vi "Update Table with Sensor Data.vi"(0 "Test Table In":string[][](table)=[["", "20"]] caption="Table", 5 "Test Data":dbl[](array[numeric]), 7 "Number of Sensors":i32=7) -> (1 "Current Elapsed":dbl format="%.2g", 2 "CountDown Time":dbl format="%.2g", 3 "CountDown Clock":picture, 4 "Test Table Out":string[][](table)=[["", "20"]] caption="Table", 8 "Test Timing Mode":enum16{"Manual", "Timed"}(ring), 14 "CountDown Text":string)   [LabVIEW 2018]
uses:
  Controls/Test Table Organization.ctl
  Timing/Controls/StateMachineStates_TEST_TDEF.ctl
panel:
  out "appended array":string[](array[string])
  out "output array":dbl[](array[numeric])
  in  "Test Data Row Documentation":T1
  out "Current Step ID":i32
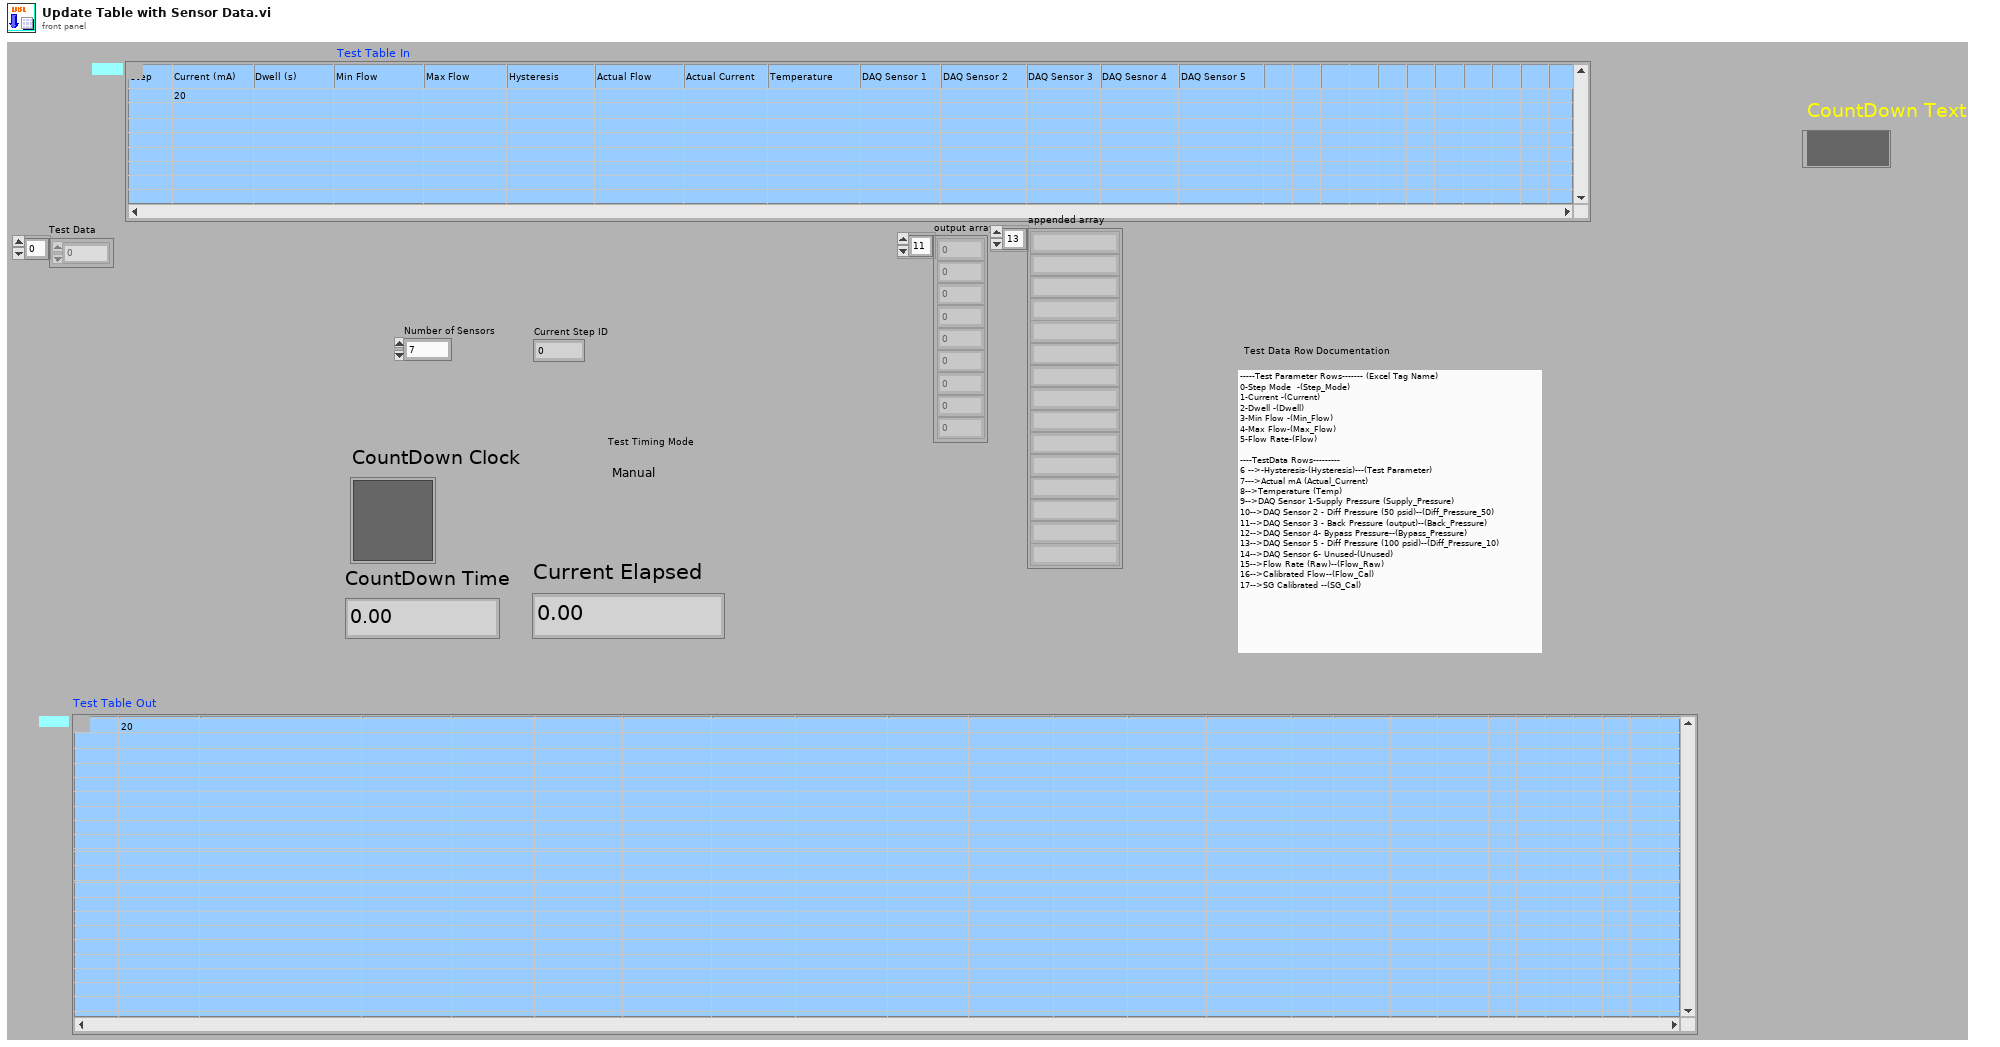
[diagram p1: front panel]
types:
  T1 = typedef "Test Table Organization.ctl" = string
  T2 = typedef "StateMachineStates_TEST_TDEF.ctl" = enum16{"Initialize", "Start", "Run Position", "Pause", "Resume", "Get Step", "Force Previous Step", "Force Next Step", "Stay on Current Step"}
  T3 = enum16{"get data", "set data", "Add Data Pair", "initialize"}
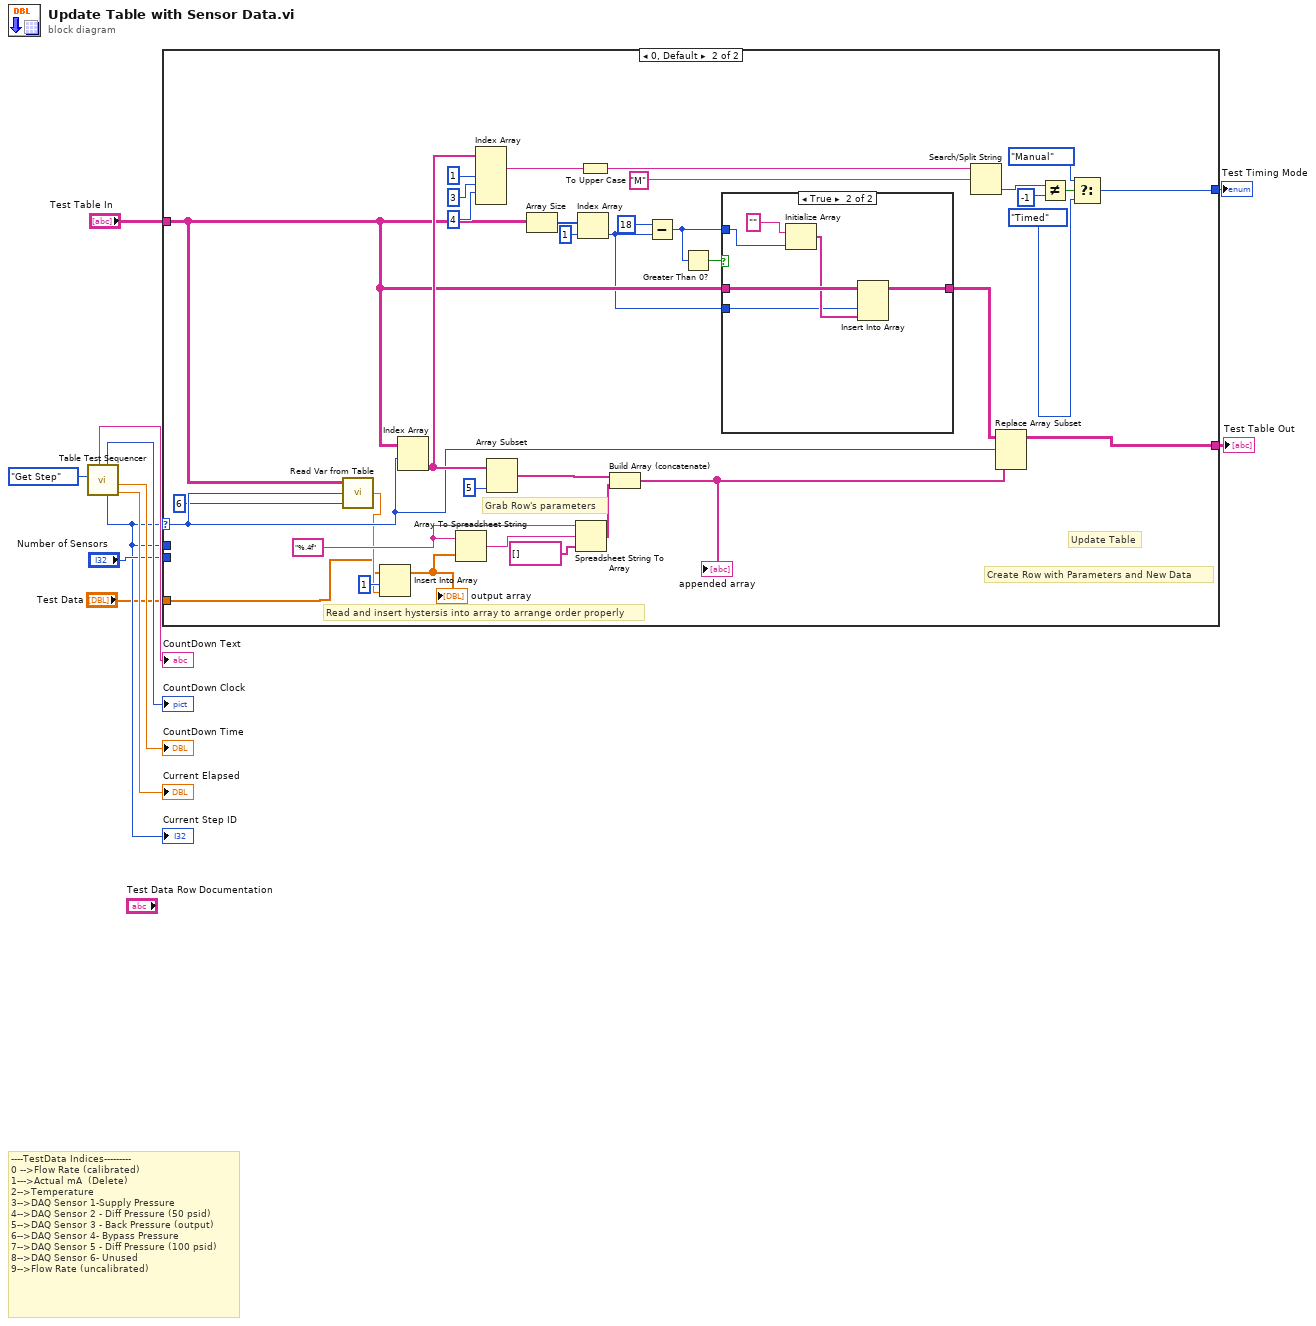
[diagram p0: block diagram]
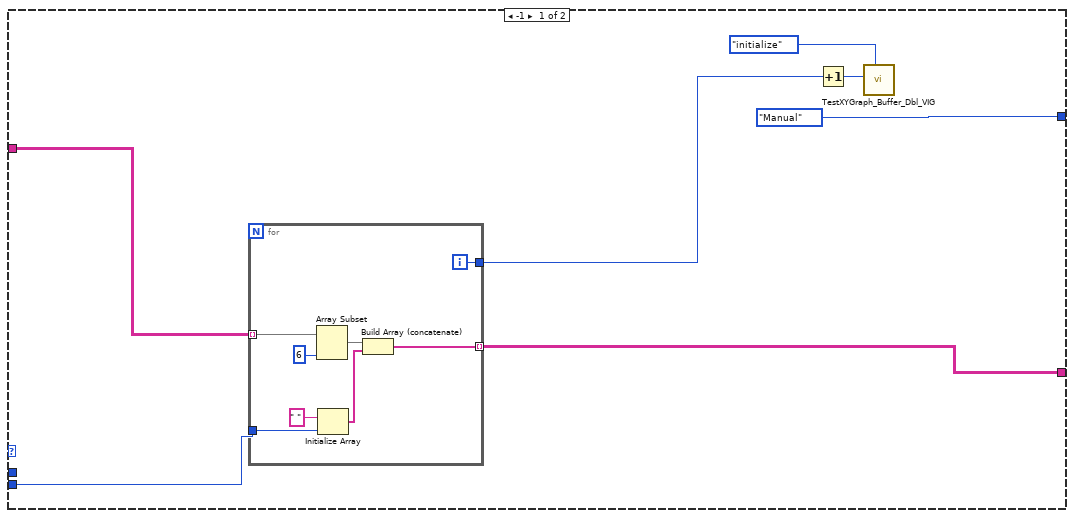
[diagram p2: hidden frame]
diagram:
  # "----TestData Indices---------\n0 -->Flow Rate (calibrated)\n1--->Actual mA  (Delete)\n2-->Temperature\n3-->DAQ Sensor 1-Supply Pressure\n4-->DAQ Sensor 2 - Diff Pressure (50 psid)\n5-->DAQ Sensor 3 - Back Pressure (output)\n6-->DAQ Sensor 4- Bypass Pressure\n7-->DAQ Sensor 5 - Diff Pressure (100 psid)\n8-->DAQ Sensor 6- Unused\n9-->Flow Rate (uncalibrated)"
  n1 = call "Table Test Sequencer.vi"("Action"=StateMachineStates_TEST_TDEF."Get Step") -> ("Current Elapsed"=→"Current Elapsed":dbl, "CountDown Time"=→"CountDown Time":dbl, "Current Step ID"=w2:i32, "CountDown Pie"=→"CountDown Clock":picture, "CountDown Text"=→"CountDown Text":string)  [unwired: 3 in, 3 out]
  "Current Step ID" <- w2
  n2 = case shown="0, Default" w2 {
    selector: w2 -> [_ w40]
    tunnel: "Number of Sensors" -> [w18 _]
    tunnel: "Test Table In" -> [w17 w31]
    tunnel: [w16 w57] -> w7
    tunnel: [enum16{"Manual", "Timed"}."Manual" ("Test Timing Mode") w47] -> w3
    tunnel: w2 -> [_ _]
    tunnel: "Test Data" -> [_ w27]
    frame -1 {
      n3 = for {
        tunnel: [w24] -> w16 mode=indexing
        tunnel: w18 -> [w22]
        tunnel: w17 -> [w21] mode=indexing
        tunnel: [w19] -> w14
        i -> [w19]
        n4 = Array Subset(array=w21, length=6 ("index")) -> (w20:string[])  [unwired: 1 in]
        n5 = Initialize Array(" " ("format string"), w22) -> (w25:string[])
        n6 = Build Array (concatenate)(w20, w25) -> (w24:string[])
      }
      n7 = Increment(x=w14) -> (x+1=w13:i32)
      n8 = call "TestXYGraph_Buffer_Dbl_VIG.vi"("Operation"=T3."initialize", "index/size"=w13) -> ()  [unwired: 8 in, 2 out]
    }
    frame 0, Default {
      w55 = "%.4f" ("format string")
      # "Update Table"
      # "Create Row with Parameters and New Data"
      # "Grab Row's parameters"
      # "Read and insert hystersis into array to arrange order properly"
      n9 = call "Read Var from Table.vi"("VAR Column Index"=6, "Current Step ID"=w40, "Value"=w31) -> ("Numeric"=w36:dbl)
      n10 = Insert Into Array(array=w27, index=1, new element=w36) -> (w38:dbl[])
      "output array" <- w38
      n11 = Index Array(array=w31, index (row)=w40) -> (element=w54:string[])  [unwired: 1 in]
      n12 = Array To Spreadsheet String(array=w38, 3:w55) -> (spreadsheet string=w60:string)  [unwired: 1 in]
      n13 = Index Array(array=w54, index #2=1 ("index"), index #3=3 ("index"), index #4=4 ("index")) -> (element #1=w53:string)  [unwired: 2 in, 4 out]
      n14 = Array Subset(array=w54, length=5 ("index")) -> (w43:string[])  [unwired: 1 in]
      n15 = Array Size(array=w31) -> (size(s)=w35:i32[])
      n16 = Spreadsheet String To Array(format string=w55, spreadsheet string=w60, array type (2D Dbl)=string[] [] ("appended array")) -> (array=w59:string[])  [unwired: 1 in]
      n17 = Index Array(array=w35, index=1) -> (element=w30:i32)
      n18 = To Upper Case(1:w53) -> (0:w52:string)
      n19 = Build Array (concatenate)(w43, w59) -> (w56:string[])
      "appended array" <- w56
      n20 = Subtract(x=18, y=w30) -> (x-y=w32:i32)
      n21 = Greater Than 0?(x=w32) -> (x > 0?=w33:bool)
      n22 = case shown="True" w33 {
        tunnel: w32 -> [_ w67]
        tunnel: w31 -> [w62 w68]
        tunnel: w30 -> [_ w64]
        tunnel: [w62 w63] -> w29
        frame False {
        }
        frame True {
          n23 = Initialize Array("" ("search string/char (-)"), w67) -> (w65:string[])
          n24 = Insert Into Array(array=w68, index (col)=w64, new element=w65) -> (w63:string[][])  [unwired: 1 in]
        }
      }
      n25 = Search/Split String(string=w52, search string/char (-)="M") -> (offset of match=w50:i32)  [unwired: 1 in, 2 out]
      n26 = Replace Array Subset(array=w29, new element=w56, index (row)=w40) -> (w57:string[][])  [unwired: 1 in]
      n27 = Not Equal?(x=w50, y=-1) -> (x != y?=w48:bool)
      n28 = Select(t=enum16{"Manual", "Timed"}."Manual" ("Test Timing Mode"), s=w48, f=enum16{"Manual", "Timed"}."Timed" ("Test Timing Mode")) -> (s? t:f=w47:enum16{"Manual", "Timed"})
    }
  }
  "Test Table Out" <- w7
  "Test Timing Mode" <- w3
